vi "INI to SQLite.vi"() -> ()   [LabVIEW 2020, in "CDM-Config.lvlib"]
uses:
  CDM-Config.lvlib
  Config-Sqlite/Config-Sqlite.lvclass
  C:/dev/lv20CE/lv-cdm/CDM-Config/Config Storage/Config Storage.lvclass
  Config-INI/Config-INI.lvclass
  Config Manager/Config Manager.lvclass
panel:
  out "error out":errorcluster
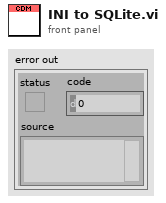
[diagram p1: front panel]
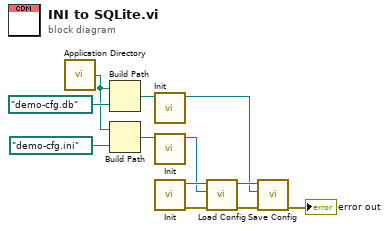
[diagram p0: block diagram]
diagram:
  n1 = call <vilib>:"Application Directory.vi"() -> ("Application Directory"=w8:path)
  n2 = Build Path(base path=w8, name or relative path=path "demo-cfg.db") -> (appended path=w9:path)
  n3 = Build Path(base path=w8, name or relative path=path "demo-cfg.ini") -> (appended path=w11:path)
  n4 = call "Init.vi"("DB Path"=w9) -> ("Config-Sqlite out"=w2:refnum<class "Config-Sqlite.lvclass">)  [unwired: 9 in, 1 out]
  n5 = call "Init.vi"("INI Path"=w11) -> ("Config-INI out"=w5:refnum<class "Config-INI.lvclass">)  [unwired: 9 in, 1 out]
  n6 = call "Init.vi"() -> ("error out"=w6:errorcluster, "Config Manager out"=w7:refnum<class "Config Manager.lvclass">)  [unwired: 10 in]
  n7 = call "Load Config.vi"("error in (no error)"=w6, "Storage"=w5, "Config Manager in"=w7) -> ("error out"=w4:errorcluster, "Config Manager out"=w3:refnum<class "Config Manager.lvclass">)  [unwired: 7 in]
  n8 = call "Save Config.vi"("error in (no error)"=w4, "Storage"=w2, "Config Manager in"=w3) -> ("error out"=→"error out":errorcluster)  [unwired: 7 in, 1 out]
